vi "SaveToFile.vi"(8 "error in":errorcluster, 10 "FileNamePrefix":string="data", 11 "TextToWrite":string) -> (0 "error out":errorcluster)   [LabVIEW 2018]
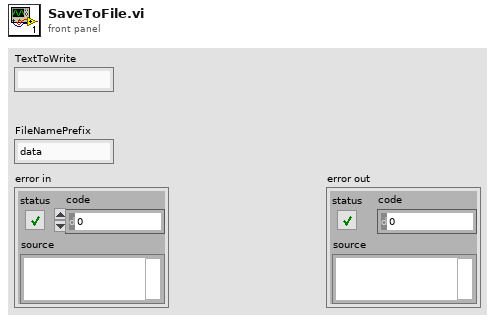
[diagram p1: front panel]
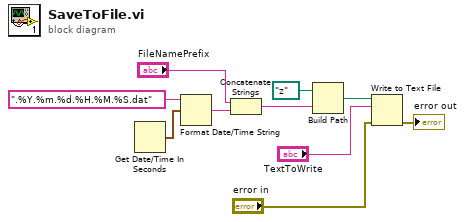
[diagram p0: block diagram]
diagram:
  n1 = Get Date/Time In Seconds() -> (seconds since 1Jan1904=w9:timestamp)
  n2 = Format Date/Time String(time format string (%c)=".%Y.%m.%d.%H.%M.%S.dat", seconds (now)=w9) -> (date/time string=w7:string)  [unwired: 1 in]
  n3 = Concatenate Strings("FileNamePrefix", w7) -> (w4:string)
  n4 = Build Path(base path=path "z:/", name or relative path=w4) -> (appended path=w2:path)
  n5 = Write to Text File(file (use dialog)=w2, text="TextToWrite", error in="error in") -> (error out=→"error out":errorcluster)  [unwired: 1 in, 2 out]
